vi "setHPADCScanRate.vi"(0 "ILCCommunications in":refnum<class "ILCCommunications.lvclass">, 5 "HPIndex":i32, 7 "WaitForTrigger":bool, 9 "TriggerIRQ":bool, 11 "error in (no error)":errorcluster) -> (4 "ILCCommunications out":refnum<class "ILCCommunications.lvclass">, 15 "error out":errorcluster)   [LabVIEW 2016, in "ILCCommunications.lvclass"]
uses:
  ILCCommunications.lvclass
  ILCCommunications.lvclass/ILCCommunications.ctl
  Common_RT_HPILC/HPILC/HPILC.lvclass
  D:/Code/ts_M1M3Support/Common_RT_ILC/ILC/ILC.lvclass
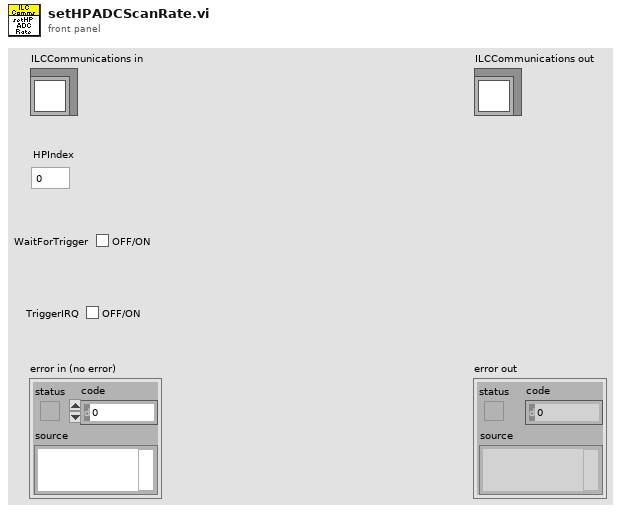
[diagram p1: front panel]
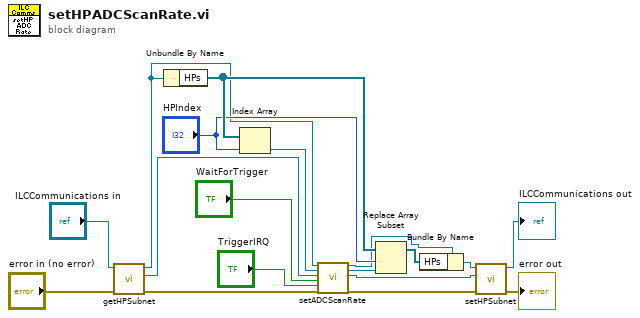
[diagram p0: block diagram]
diagram:
  n1 = call "getHPSubnet.vi"("error in (no error)"="error in (no error)", "ILCCommunications in"="ILCCommunications in") -> ("error out"=w2:errorcluster, "Modbus"=w10:refnum<class "IModbus.lvclass">, "ILCCommunications out"=w4:refnum<class "ILCCommunications.lvclass">)  [unwired: 7 in]
  n2 = Unbundle By Name(w4) -> ("HPs"=w18:refnum<class "HPILC.lvclass">[])
  n3 = Index Array(array=w18, index="HPIndex") -> (element=w11:refnum<class "HPILC.lvclass">)
  n4 = call "setADCScanRate.vi"("ILCCommunications in"=w4, "ILC in"=w11, "Modbus in"=w10, "WaitForTrigger"="WaitForTrigger", "TriggerIRQ"="TriggerIRQ", "error in (no error)"=w2) -> ("ILCCommunications out"=w3:refnum<class "ILCCommunications.lvclass">, "ILC out"=w8:refnum<class "HPILC.lvclass">, "Modbus out"=w9:refnum<class "IModbus.lvclass">, "error out"=w1:errorcluster)  [unwired: 10 in]
  n5 = Replace Array Subset(array=w18, new element=w8, index="HPIndex") -> (w17:refnum<class "HPILC.lvclass">[])
  n6 = Bundle By Name(cluster=w3, "HPs"=w17) -> (w13:refnum<class "ILCCommunications.lvclass">)
  n7 = call "setHPSubnet.vi"("error in (no error)"=w1, "Modbus"=w9, "ILCCommunications in"=w13) -> ("error out"=→"error out":errorcluster, "ILCCommunications out"=→"ILCCommunications out":refnum<class "ILCCommunications.lvclass">)  [unwired: 7 in]
